vi "Percent of Full Screen in Pixels.vi"(8 "error in (no error)":errorcluster, 11 "Percent of Screen(%)":dbl) -> (0 "error out":errorcluster, 2 "Y":i16, 3 "X":i16)   [LabVIEW 2014]
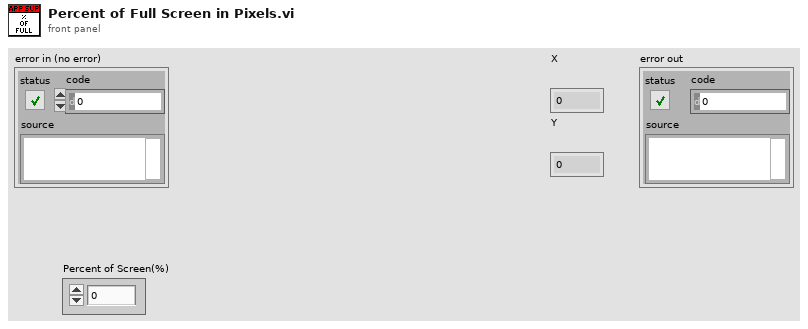
[diagram p1: front panel]
types:
  T1 = typedef "LVRectTypeDef.ctl" = cluster{"Left":i16, "Top":i16, "Right":i16, "Bottom":i16}
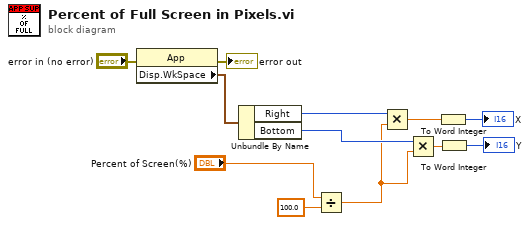
[diagram p0: block diagram]
diagram:
  n1 = property class="App"(error in="error in (no error)") -> (error out=→"error out":errorcluster, "Disp.WkSpace"=w12:T1)  [unwired: 1 in, 1 out]
  n2 = Unbundle By Name(w12) -> ("Right"=w9:i16, "Bottom"=w8:i16)
  n3 = Divide(x="Percent of Screen(%)", y=100.0) -> (x/y=w1:dbl)
  n4 = Multiply(x=w9, y=w1) -> (x*y=w7:dbl)
  n5 = Multiply(x=w8, y=w1) -> (x*y=w6:dbl)
  n6 = To Word Integer(number=w7) -> (16bit integer=→"X":i16)
  n7 = To Word Integer(number=w6) -> (16bit integer=→"Y":i16)
